vi "ParsesDATA.vi"(11 "ZCANDataObj":T1[](array[typedef])) -> (3 "ZCANDataObj(out)":T1[](array[typedef]), 4 "CAN报文显示":string[][](table))   [LabVIEW 2018]
uses:
  data_type/ZCANDataObj.ctl
panel:
  in  "列表索引0是最新的报文? (T)":bool=TRUE
  in  "最大显示帧数(100)":i32=100
  in  "空数组":u8[](array[numeric])
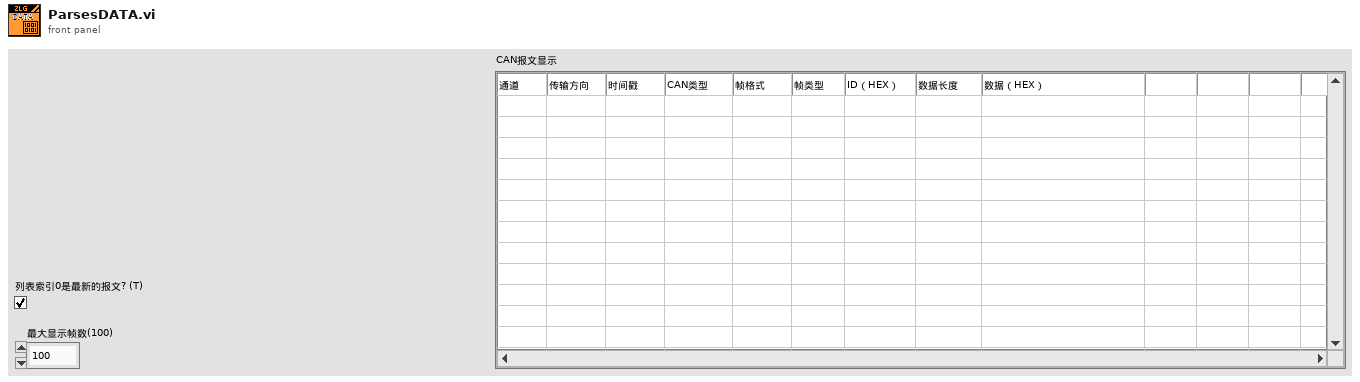
[diagram p1: front panel]
types:
  T1 = typedef "ZCANDataObj.ctl" = cluster{"数据类型":u8, "CAN通道号":u8, "rawVal(未使用)":u16, "extraData[4]（未使用）":cluster{"[0]":u8, "[1]":u8, "[2]":u8, "[3]":u8}, "canCANFDData":cluster{"时间戳+混合标志位":cluster{"时间戳":u64, "混合标志位":u32}, "extraData[4]（未使用）":cluster{"[0]":u8, "[1]":u8, "[2]":u8, "[3]":u8}, "frame":cluster{"can_id":u32, "数据长度":u8, "CANFD加速？":u8, "__res0":u8, "__res1":u8, "data":cluster{"CAN数据[0]":u8, "CAN数据[1]":u8, "CAN数据[2]":u8, "CAN数据[3]":u8, "CAN数据[4]":u8, "CAN数据[5]":u8, "CAN数据[6]":u8, "CAN数据[7]":u8, "CAN数据[8]":u8, "CAN数据[9]":u8, "CAN数据[10]":u8, "CAN数据[11] ":u8, "CAN数据[12] ":u8, "CAN数据[13] ":u8, "CAN数据[14] ":u8, "CAN数据[15] ":u8, "CAN数据[16]":u8, "CAN数据[17]":u8, "CAN数据[18]":u8, "CAN数据[19]":u8, "CAN数据[20]":u8, "CAN数据[21]":u8, "CAN数据[22]":u8, "CAN数据[23]":u8, "CAN数据[24] ":u8, "CAN数据[25]":u8, "CAN数据[26]":u8, "CAN数据[27]":u8, "CAN数据[28]":u8, "CAN数据[29]":u8, "CAN数据[30]":u8, "CAN数据[31]":u8, "CAN数据[32]":u8, "CAN数据[33]":u8, "CAN数据[34]":u8, "CAN数据[35]":u8, "CAN数据[36]":u8, "CAN数据[37]":u8, "CAN数据[38]":u8, "CAN数据[39]":u8, "CAN数据[40]":u8, "CAN数据[41]":u8, "CAN数据[42]":u8, "CAN数据[43]":u8, "CAN数据[44]":u8, "CAN数据[45]":u8, "CAN数据[46]":u8, "CAN数据[47]":u8, "CAN数据[48]":u8, "CAN数据[49]":u8, "CAN数据[50]":u8, "CAN数据[51]":u8, "CAN数据[52]":u8, "CAN数据[53]":u8, "CAN数据[54]":u8, "CAN数据[55]":u8, "CAN数据[56]":u8, "CAN数据[57]":u8, "CAN数据[58]":u8, "CAN数据[59]":u8, "CAN数据[60]":u8, "CAN数据[61]":u8, "CAN数据[62]":u8, "CAN数据[63]":u8}}}, "raw[92]（未使用）":cluster{"[0]":u8, "[1]":u8, "[2]":u8, "[3]":u8, "[4]":u8, "[5]":u8, "[6]":u8, "[7]":u8, "[8]":u8, "[9]":u8, "[10]":u8, "[11]":u8, "[12]":u8, "[13]":u8, "[14]":u8, "[15]":u8, "[16]":u8, "[17]":u8, "[18]":u8, "[19]":u8, "[20]":u8, "[21]":u8, "[22]":u8, "[23]":u8, "[24]":u8, "[25]":u8, "[26]":u8, "[27]":u8, "[28]":u8, "[29]":u8, "[30]":u8, "[31]":u8, "[32]":u8, "[33]":u8, "[34]":u8, "[35]":u8, "[36]":u8, "[37]":u8, "[38]":u8, "[39]":u8, "[40]":u8, "[41]":u8, "[42]":u8, "[43]":u8, "[44]":u8, "[45]":u8, "[46]":u8, "[47]":u8, "[48]":u8, "[49]":u8, "[50]":u8, "[51]":u8, "[52]":u8, "[53]":u8, "[54]":u8, "[55]":u8, "[56]":u8, "[57]":u8, "[58]":u8, "[59]":u8, "[60]":u8, "[61]":u8, "[62]":u8, "[63]":u8, "[64]":u8, "[65]":u8, "[73]":u8, "[72]":u8, "[71]":u8, "[70]":u8, "[69]":u8, "[68]":u8, "[67]":u8, "[66]":u8, "[74]":u8, "[75]":u8, "[83]":u8, "[82]":u8, "[81]":u8, "[80]":u8, "[79]":u8, "[78]":u8, "[77]":u8, "[76]":u8, "[84]":u8, "[85]":u8, "[91]":u8, "[90]":u8, "[89]":u8, "[88]":u8, "[87]":u8, "[86]":u8}}
  T2 = cluster{"时间戳+混合标志位":cluster{"时间戳":u64, "混合标志位":u32}, "extraData[4]（未使用）":cluster{"[0]":u8, "[1]":u8, "[2]":u8, "[3]":u8}, "frame":cluster{"can_id":u32, "数据长度":u8, "CANFD加速？":u8, "__res0":u8, "__res1":u8, "data":cluster{"CAN数据[0]":u8, "CAN数据[1]":u8, "CAN数据[2]":u8, "CAN数据[3]":u8, "CAN数据[4]":u8, "CAN数据[5]":u8, "CAN数据[6]":u8, "CAN数据[7]":u8, "CAN数据[8]":u8, "CAN数据[9]":u8, "CAN数据[10]":u8, "CAN数据[11] ":u8, "CAN数据[12] ":u8, "CAN数据[13] ":u8, "CAN数据[14] ":u8, "CAN数据[15] ":u8, "CAN数据[16]":u8, "CAN数据[17]":u8, "CAN数据[18]":u8, "CAN数据[19]":u8, "CAN数据[20]":u8, "CAN数据[21]":u8, "CAN数据[22]":u8, "CAN数据[23]":u8, "CAN数据[24] ":u8, "CAN数据[25]":u8, "CAN数据[26]":u8, "CAN数据[27]":u8, "CAN数据[28]":u8, "CAN数据[29]":u8, "CAN数据[30]":u8, "CAN数据[31]":u8, "CAN数据[32]":u8, "CAN数据[33]":u8, "CAN数据[34]":u8, "CAN数据[35]":u8, "CAN数据[36]":u8, "CAN数据[37]":u8, "CAN数据[38]":u8, "CAN数据[39]":u8, "CAN数据[40]":u8, "CAN数据[41]":u8, "CAN数据[42]":u8, "CAN数据[43]":u8, "CAN数据[44]":u8, "CAN数据[45]":u8, "CAN数据[46]":u8, "CAN数据[47]":u8, "CAN数据[48]":u8, "CAN数据[49]":u8, "CAN数据[50]":u8, "CAN数据[51]":u8, "CAN数据[52]":u8, "CAN数据[53]":u8, "CAN数据[54]":u8, "CAN数据[55]":u8, "CAN数据[56]":u8, "CAN数据[57]":u8, "CAN数据[58]":u8, "CAN数据[59]":u8, "CAN数据[60]":u8, "CAN数据[61]":u8, "CAN数据[62]":u8, "CAN数据[63]":u8}}}
  T3 = cluster{"can_id":u32, "数据长度":u8, "CANFD加速？":u8, "__res0":u8, "__res1":u8, "data":cluster{"CAN数据[0]":u8, "CAN数据[1]":u8, "CAN数据[2]":u8, "CAN数据[3]":u8, "CAN数据[4]":u8, "CAN数据[5]":u8, "CAN数据[6]":u8, "CAN数据[7]":u8, "CAN数据[8]":u8, "CAN数据[9]":u8, "CAN数据[10]":u8, "CAN数据[11] ":u8, "CAN数据[12] ":u8, "CAN数据[13] ":u8, "CAN数据[14] ":u8, "CAN数据[15] ":u8, "CAN数据[16]":u8, "CAN数据[17]":u8, "CAN数据[18]":u8, "CAN数据[19]":u8, "CAN数据[20]":u8, "CAN数据[21]":u8, "CAN数据[22]":u8, "CAN数据[23]":u8, "CAN数据[24] ":u8, "CAN数据[25]":u8, "CAN数据[26]":u8, "CAN数据[27]":u8, "CAN数据[28]":u8, "CAN数据[29]":u8, "CAN数据[30]":u8, "CAN数据[31]":u8, "CAN数据[32]":u8, "CAN数据[33]":u8, "CAN数据[34]":u8, "CAN数据[35]":u8, "CAN数据[36]":u8, "CAN数据[37]":u8, "CAN数据[38]":u8, "CAN数据[39]":u8, "CAN数据[40]":u8, "CAN数据[41]":u8, "CAN数据[42]":u8, "CAN数据[43]":u8, "CAN数据[44]":u8, "CAN数据[45]":u8, "CAN数据[46]":u8, "CAN数据[47]":u8, "CAN数据[48]":u8, "CAN数据[49]":u8, "CAN数据[50]":u8, "CAN数据[51]":u8, "CAN数据[52]":u8, "CAN数据[53]":u8, "CAN数据[54]":u8, "CAN数据[55]":u8, "CAN数据[56]":u8, "CAN数据[57]":u8, "CAN数据[58]":u8, "CAN数据[59]":u8, "CAN数据[60]":u8, "CAN数据[61]":u8, "CAN数据[62]":u8, "CAN数据[63]":u8}}
  T4 = cluster{"CAN数据[0]":u8, "CAN数据[1]":u8, "CAN数据[2]":u8, "CAN数据[3]":u8, "CAN数据[4]":u8, "CAN数据[5]":u8, "CAN数据[6]":u8, "CAN数据[7]":u8, "CAN数据[8]":u8, "CAN数据[9]":u8, "CAN数据[10]":u8, "CAN数据[11] ":u8, "CAN数据[12] ":u8, "CAN数据[13] ":u8, "CAN数据[14] ":u8, "CAN数据[15] ":u8, "CAN数据[16]":u8, "CAN数据[17]":u8, "CAN数据[18]":u8, "CAN数据[19]":u8, "CAN数据[20]":u8, "CAN数据[21]":u8, "CAN数据[22]":u8, "CAN数据[23]":u8, "CAN数据[24] ":u8, "CAN数据[25]":u8, "CAN数据[26]":u8, "CAN数据[27]":u8, "CAN数据[28]":u8, "CAN数据[29]":u8, "CAN数据[30]":u8, "CAN数据[31]":u8, "CAN数据[32]":u8, "CAN数据[33]":u8, "CAN数据[34]":u8, "CAN数据[35]":u8, "CAN数据[36]":u8, "CAN数据[37]":u8, "CAN数据[38]":u8, "CAN数据[39]":u8, "CAN数据[40]":u8, "CAN数据[41]":u8, "CAN数据[42]":u8, "CAN数据[43]":u8, "CAN数据[44]":u8, "CAN数据[45]":u8, "CAN数据[46]":u8, "CAN数据[47]":u8, "CAN数据[48]":u8, "CAN数据[49]":u8, "CAN数据[50]":u8, "CAN数据[51]":u8, "CAN数据[52]":u8, "CAN数据[53]":u8, "CAN数据[54]":u8, "CAN数据[55]":u8, "CAN数据[56]":u8, "CAN数据[57]":u8, "CAN数据[58]":u8, "CAN数据[59]":u8, "CAN数据[60]":u8, "CAN数据[61]":u8, "CAN数据[62]":u8, "CAN数据[63]":u8}
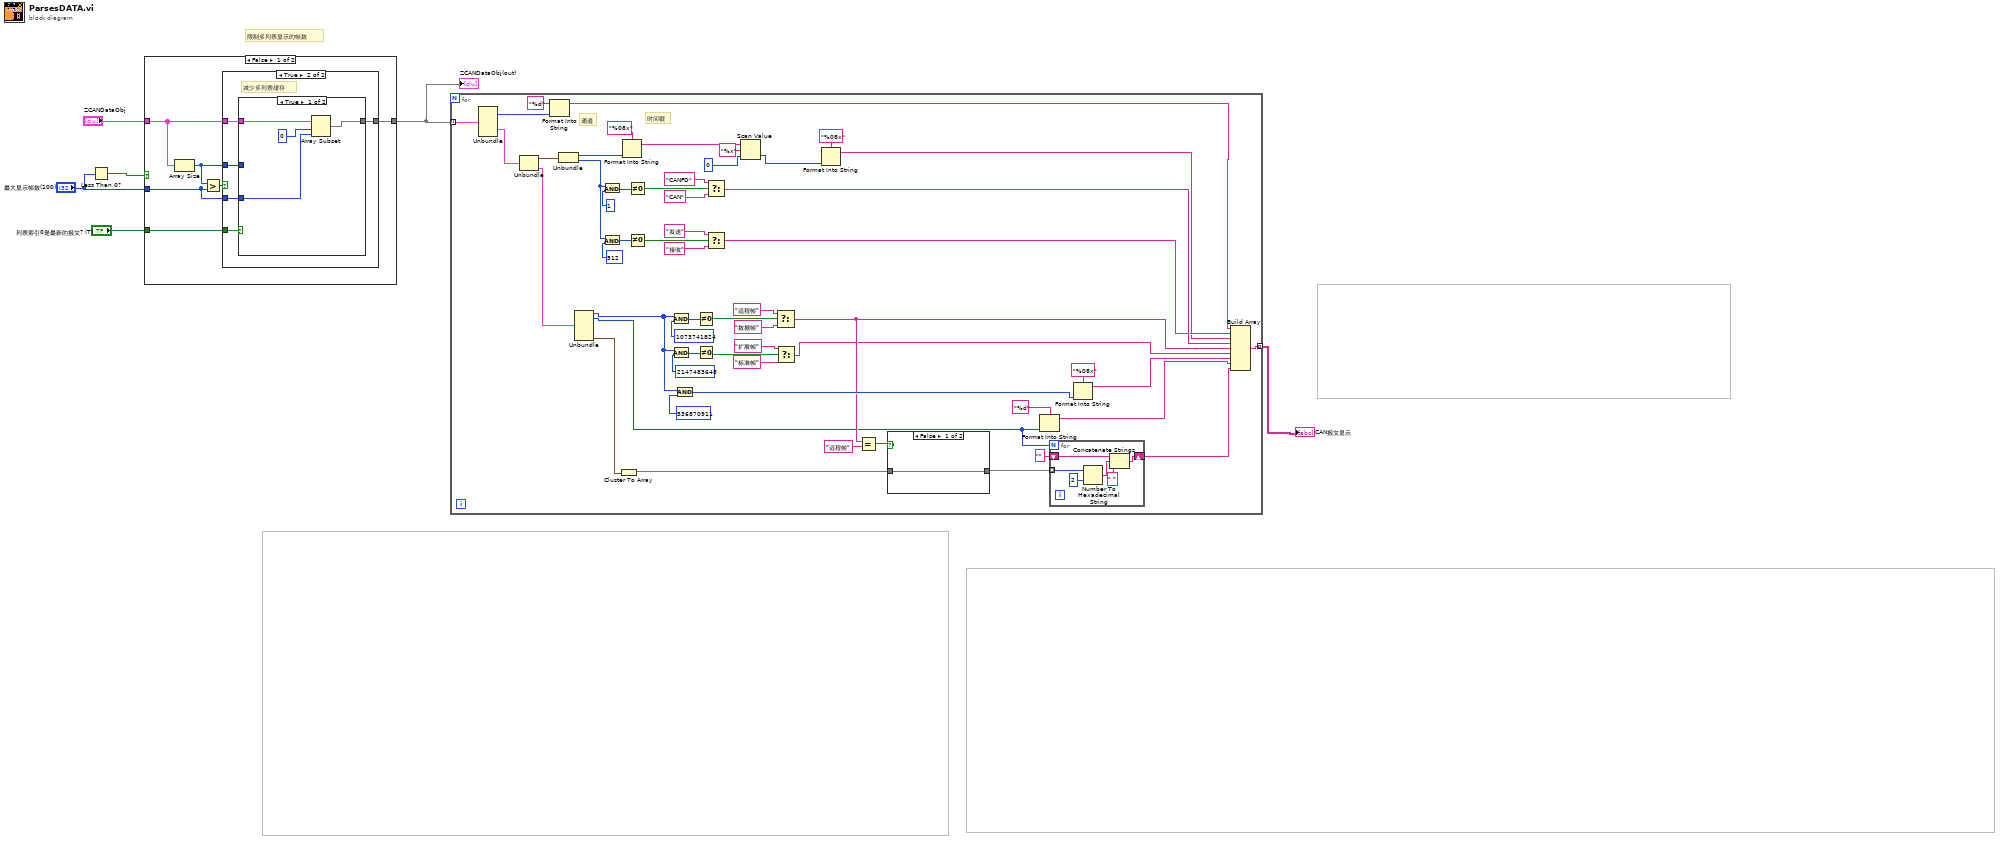
[diagram p0: block diagram]
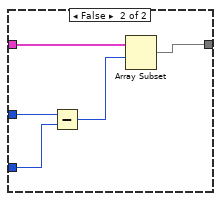
[diagram p3: hidden frame]
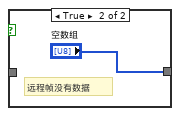
[diagram p5: hidden frame]
diagram:
  # "限制多列表显示的帧数"
  n1 = Less Than 0?(x="最大显示帧数(100)") -> (x < 0?=w3:bool)
  n2 = case shown="False" w3 {
    tunnel: "ZCANDataObj" -> [w11 w28]
    tunnel: [w10 w28] -> w1
    tunnel: "列表索引0是最新的报文? (T)" -> [w9 _]
    tunnel: "最大显示帧数(100)" -> [w7 _]
    frame False {
      n3 = Array Size(array=w11) -> (size(s)=w8:i32)
      n4 = Greater?(x=w8, y=w7) -> (0:w12:bool)
      n5 = case shown="True" w12 {
        tunnel: w11 -> [w13 w18]
        tunnel: [w13 w17] -> w10
        tunnel: w7 -> [_ w16]
        tunnel: w9 -> [_ w15]
        tunnel: w8 -> [_ w14]
        frame False {
          # "Size is not too big don't trim it"
        }
        frame True {
          # "减少多列表缓存"
          n6 = case shown="True" w15 {
            tunnel: w18 -> [w22 w27]
            tunnel: [w21 w26] -> w17
            tunnel: w16 -> [w19 w24]
            tunnel: w14 -> [_ w25]
            frame True {
              n7 = Array Subset(array=w22, index=0, length=w19) -> (w21:T1[])
            }
            frame False {
              n8 = Subtract(x=w25, y=w24) -> (x-y=w23:i32)
              n9 = Array Subset(array=w27, index=w23) -> (w26:T1[])  [unwired: 1 in]
            }
          }
        }
      }
    }
    frame True {
      # "-1 means don't limit the size of the array"
    }
  }
  "ZCANDataObj(out)" <- w1
  n10 = for {
    tunnel: w1 -> [w64] mode=indexing
    tunnel: [w68] -> w6 mode=indexing
    # "时间戳"
    # "通道"
    n11 = Unbundle(w64) -> ("CAN通道号"=w62:u8, "canCANFDData"=w60:T2)  [unwired: 4 out]
    n12 = Unbundle(w60) -> ("时间戳+混合标志位"=w59:cluster{"时间戳":u64, "混合标志位":u32}, "frame"=w44:T3)  [unwired: 1 out]
    n13 = Format Into String(format string="%d", w62) -> (resulting string=w61:string)  [unwired: 2 in, 1 out]
    n14 = Unbundle(w59) -> ("时间戳"=w36:u64, "混合标志位"=w46:u32)
    n15 = Unbundle(w44) -> ("can_id"=w43:u32, "数据长度"=w29:u8, "data"=w42:T4)  [unwired: 3 out]
    n16 = And(x=w46, y=u32 1) -> (x .and. y?=w56:u32)
    n17 = And(x=w46, y=u32 512) -> (x .and. y?=w50:u32)
    n18 = Cluster To Array(cluster=w42) -> (array=w71:u8[])
    n19 = Format Into String(format string="%08x", w36) -> (resulting string=w35:string)  [unwired: 2 in, 1 out]
    n20 = Not Equal To 0?(x=w56) -> (x != 0?=w53:bool)
    n21 = Not Equal To 0?(x=w50) -> (x != 0?=w47:bool)
    n22 = And(x=w43, y=u32 1073741824) -> (x .and. y?=w80:u32)
    n23 = And(x=w43, y=u32 2147483648) -> (x .and. y?=w81:u32)
    n24 = And(x=w43, y=u32 536870911) -> (x .and. y?=w65:u32)
    n25 = Not Equal To 0?(x=w80) -> (x != 0?=w75:bool)
    n26 = Not Equal To 0?(x=w81) -> (x != 0?=w74:bool)
    n27 = Select(t="CANFD", s=w53, f="CAN") -> (s? t:f=w52:string)
    n28 = Select(t="发送", s=w47, f="接收") -> (s? t:f=w45:string)
    n29 = Scan Value(string=w35, format string="%x", default (0 dbl)=0) -> (value=w31:i32)  [unwired: 1 out]
    n30 = Select(t="远程帧", s=w75, f="数据帧") -> (s? t:f=w41:string)
    n31 = Select(t="扩展帧", s=w74, f="标准帧") -> (s? t:f=w40:string)
    n32 = Format Into String(format string="%08x", w31) -> (resulting string=w30:string)  [unwired: 2 in, 1 out]
    n33 = Equal?(x=w41, y="远程帧") -> (x = y?=w72:bool)
    n34 = case shown="False" w72 {
      tunnel: [w91 "空数组"] -> w66
      tunnel: w71 -> [w91 _]
      frame False {
      }
      frame True {
        # "远程帧没有数据"
      }
    }
    n35 = Format Into String(format string="%d", w29) -> (resulting string=w38:string)  [unwired: 2 in, 1 out]
    n36 = for {
      N: w29 -> [_]
      shift-right: [w87] -> w37
      shift-left: "" -> [w85]
      tunnel: w66 -> [w86] mode=indexing
      n37 = Number To Hexadecimal String(1:i16 2 ("width (-)"), 2:w86) -> (0:w89:string)
      n38 = Concatenate Strings(w85, w89, " " ("string")) -> (w87:string)
    }
    n39 = Format Into String(format string="%08x", w65) -> (resulting string=w39:string)  [unwired: 2 in, 1 out]
    n40 = Build Array(w61, w45, w30, w52, w41, w40, w39, w38, w37) -> (w68:string[])
  }
  "CAN报文显示" <- w6
